vi "Convert_AC_PctVolt.vi"(1 "AC_Volt%":dbl) -> (0 "AC_Volt":dbl[unit])   [LabVIEW 2024]
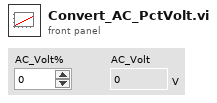
[diagram p1: front panel]
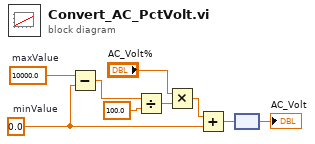
[diagram p0: block diagram]
diagram:
  w6 = 10000.0  # maxValue
  w3 = 0.0  # minValue
  n1 = Subtract(x=w6, y=w3) -> (x-y=w5:dbl)
  n2 = Divide(x=w5, y=100.0) -> (x/y=w4:dbl)
  n3 = Multiply(x="AC_Volt%", y=w4) -> (x*y=w9:dbl)
  n4 = Add(x=w9, y=w3) -> (x+y=w8:dbl)
  n5 = node(w8) -> (→"AC_Volt":dbl[unit])
